vi "BLE_r&w.vi"() -> ()   [LabVIEW 2020]
uses:
  D:/Project/LabView/LabVIEW-BLE-Driver-main/BLE_base/BLELib.dll
  BLELib.dll
panel:
  out "错误输出":errorcluster
  out "StopResult":string
  out "添加的数组":u32[](array[numeric])
  out "NotifyResult":string
  out "Watcher Response":string
  in  "停止接收Notify":bool
  out "WriteResult":string
  out "NotifyStartResult":string
  out "目标设备地址":string
  in  "停止搜寻":bool
  out "蓝牙设备地址列表":string[][](array[string])
  out "设备搜寻状态":string
  in  "是否开启BLE蓝牙log日志":bool
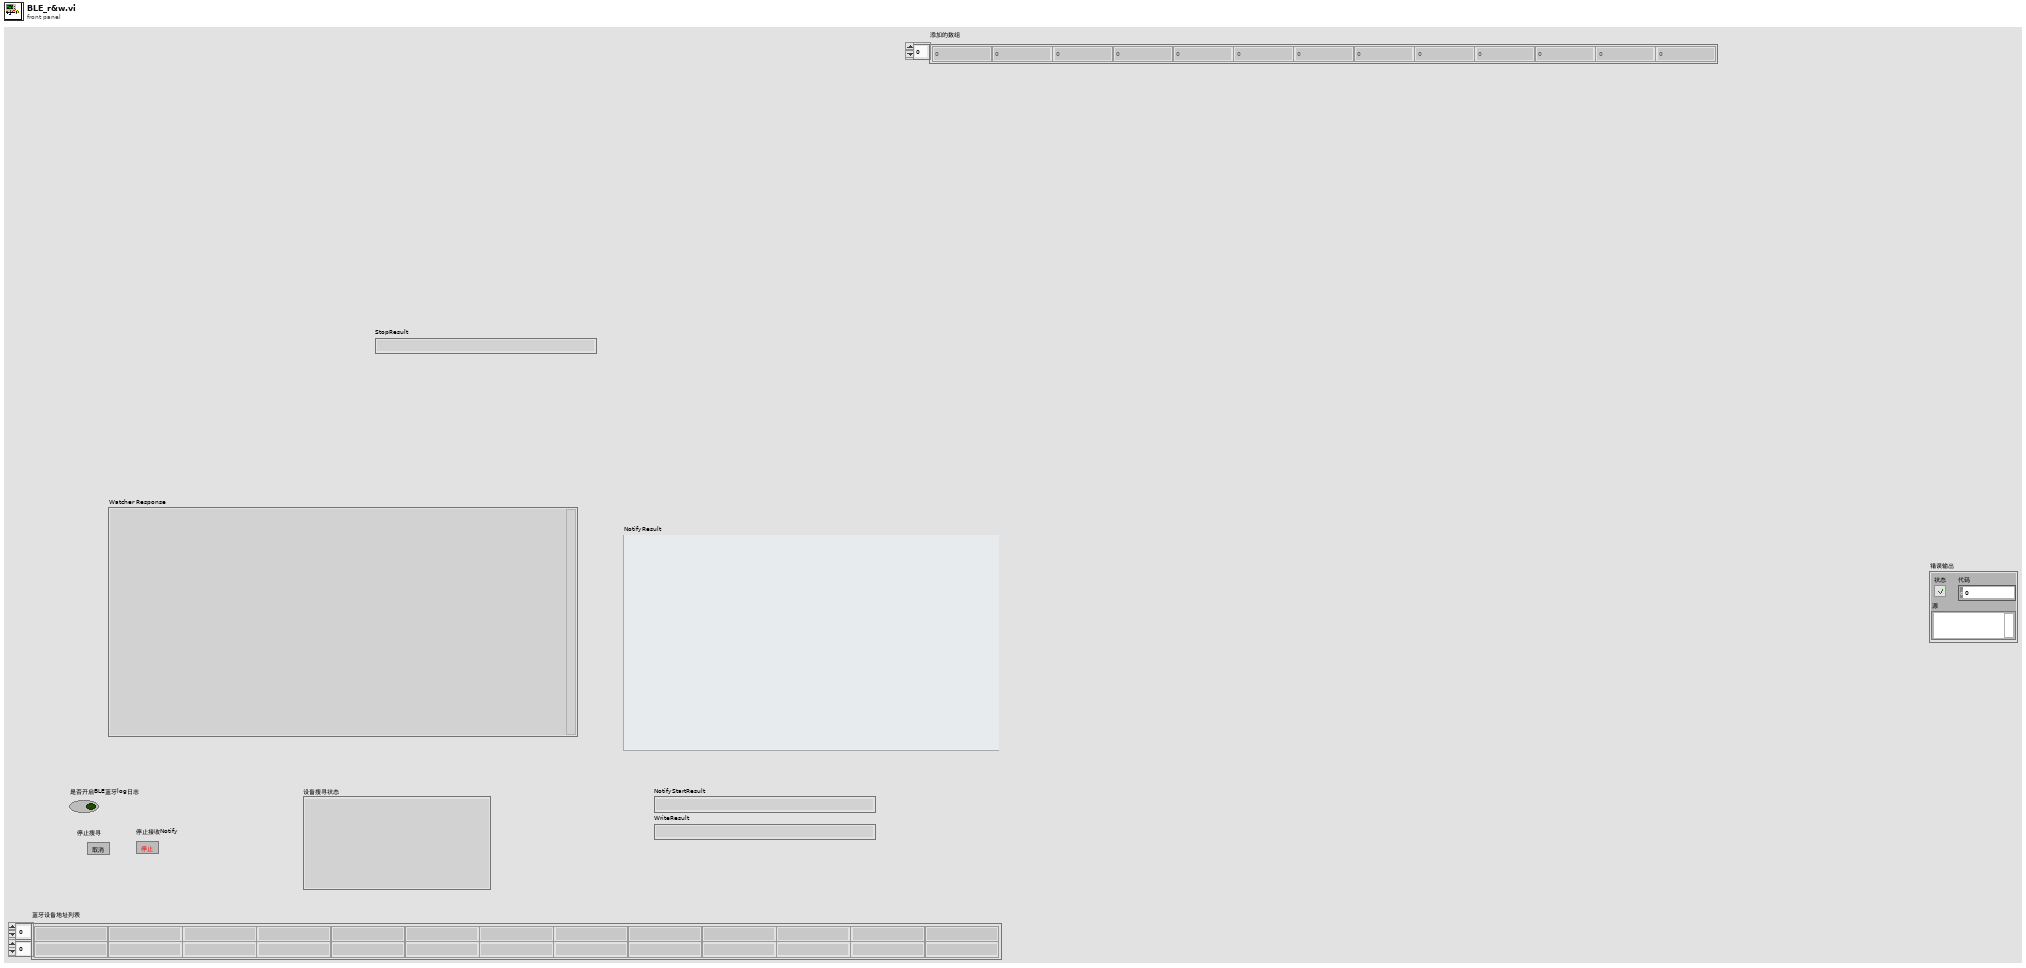
[diagram p1: front panel]
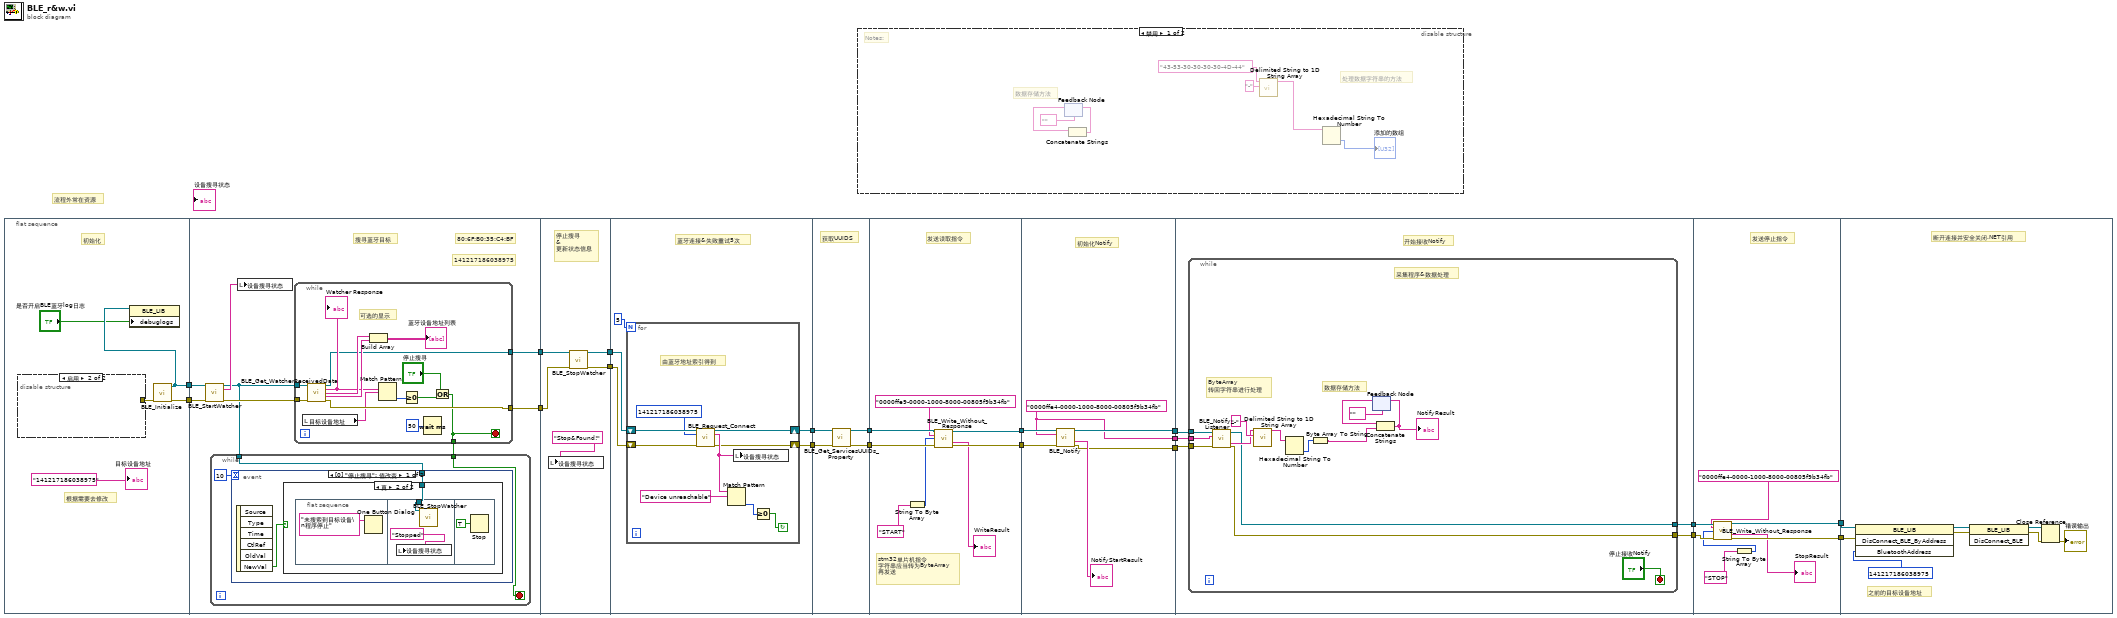
[diagram p0: block diagram]
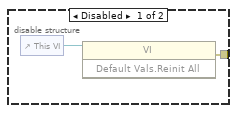
[diagram p3: hidden frame]
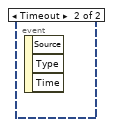
[diagram p5: hidden frame]
diagram:
  # "流程外常在资源"
  n1 = flat-sequence {
    tunnel: [w23] -> w19
    tunnel: [w21] -> w18
    tunnel: w19 -> [w34]
    tunnel: w18 -> [w33]
    tunnel: [w31] -> w17
    tunnel: [w30] -> w16
    tunnel: w17 -> [w62]
    tunnel: w16 -> [w60]
    tunnel: [w61] -> w15
    tunnel: [w59] -> w14
    tunnel: w15 -> [w67]
    tunnel: w14 -> [w66]
    tunnel: [w65] -> w13
    tunnel: [w64] -> w12
    tunnel: w13 -> [w81]
    tunnel: w12 -> [w80]
    tunnel: [w79] -> w11
    tunnel: [w78] -> w9
    tunnel: w11 -> [w89]
    tunnel: [w88] -> w10
    tunnel: w9 -> [w86]
    tunnel: [w87] -> w8
    tunnel: w10 -> [w95]
    tunnel: w8 -> [w94]
    tunnel: [w92] -> w7
    tunnel: [w91] -> w6
    tunnel: [w90] -> w5
    tunnel: w7 -> [w100]
    tunnel: w6 -> [w99]
    tunnel: w5 -> [w98]
    tunnel: [w97] -> w4
    tunnel: [w96] -> w3
    tunnel: w4 -> [w122]
    tunnel: w3 -> [w121]
    tunnel: [w117] -> w2
    tunnel: [w116] -> w1
    tunnel: w2 -> [w130]
    tunnel: w1 -> [w129]
    frame #0 {
      # "根据需要去修改"
      # "初始化"
      n2 = disable-structure shown="启用" {
        disable-tunnel: [w25 _] -> w24
        frame Disabled {
          n3 = control-ref of="This VI"() -> (w26:refnum<vi>)
          n4 = invoke class="VI" method="Default Vals.Reinit All"(reference=w26) -> (error out=w25:errorcluster)  [unwired: 2 in, 2 out]
        }
        frame Enabled {
        }
      }
      n5 = call "BLE_Initialize.vi"("error in (no error)"=w24) -> (".NET Refnum out"=w23:refnum<k24>, "error out"=w21:errorcluster)  [unwired: 13 in]
      n6 = property class="BLE_LIB"(reference=w23, "debuglogs"="是否开启BLE蓝牙log日志") -> ()  [unwired: 1 in, 2 out]
      "目标设备地址" <- "141217186038975" ("正则表达式")
    }
    frame #1 {
      # "141217186038975"
      # "80:6F:B0:35:C4:BF"
      # "搜寻蓝牙目标"
      n7 = call "BLE_StartWatcher.vi"(".NET Refnum in"=w34, "error in (no error)"=w33) -> (".NET Refnum out"=w28:refnum<k24>, "StartDeviceWatcher"=w29:string, "error out"=w32:errorcluster)  [unwired: 11 in]
      n8 = local write "设备搜寻状态"(w29) -> ()
      n9 = while {
        tunnel: w28 -> [w58]
        tunnel: w32 -> [w57]
        tunnel: [w49] -> w31
        tunnel: [w48] -> w30
        tunnel: [w46] -> w27
        stop <- w46 stop-if-true
        # "可选的显示"
        n10 = local read "目标设备地址"() -> (w47:string)
        n11 = call "BLE_Get_WatcherReceivedData.vi"(".NET Refnum in"=w58, "error in (no error)"=w57) -> (".NET Refnum out"=w49:refnum<k24>, "Watcher Response"=w53:string, "Bluetooth Addr"=w56:string[], "Bluetooth Raw Addr"=w55:string[], "error out"=w48:errorcluster)  [unwired: 6 in, 3 out]
        "Watcher Response" <- w53
        n12 = Build Array(w56, w55) -> (→"蓝牙设备地址列表":string[][])
        n13 = Match Pattern(string=w53, regular expression=w47) -> (offset past match=w52:i32)  [unwired: 1 in, 3 out]
        n14 = Greater Or Equal To 0?(x=w52) -> (x >= 0?=w51:bool)
        n15 = Wait (ms)(milliseconds to wait=u32 50 ("等待时间（毫秒）")) -> ()  [unwired: 1 out]
        n16 = Or(x="停止搜寻", y=w51) -> (x .or. y?=w46:bool)
      }
      n17 = while {
        tunnel: w28 -> [w37]
        tunnel: w27 -> [w36]
        stop <- w36 stop-if-true
        n18 = event shown="[0] \"停止搜寻\": 值改变" {
          selector: _ -> [_ _]
          dyn-events: _ -> [_ _]
          timeout: 10 -> [_ _]
          tunnel: w37 -> [w39 _]
          event "停止搜寻": Value Change {
            n19 = event-data() -> ("NewVal"=w38:bool)  [unwired: 1 in, 5 out]
            n20 = case shown="真" w38 {
              tunnel: w39 -> [_ w40]
              frame False {
              }
              frame True {
                n21 = flat-sequence {
                  tunnel: w40 -> [w43]
                  frame #0 {
                    n22 = One Button Dialog(message="未搜索到目标设备\n程序停止" ("消息")) -> ()  [unwired: 1 in, 1 out]
                  }
                  frame #1 {
                    n23 = local write "设备搜寻状态"("Stopped") -> ()
                    n24 = call "BLE_StopWatcher.vi"(".NET Refnum in"=w43) -> ()  [unwired: 12 in, 3 out]
                  }
                  frame #2 {
                    n25 = Stop(stop? (T)=TRUE ("停止？(T)")) -> ()
                  }
                }
              }
            }
          }
          event Timeout {
            n26 = event-data() -> ()  [unwired: 1 in, 3 out]
          }
        }
      }
    }
    frame #2 {
      # "停止搜寻\n&\n更新状态信息"
      n27 = local write "设备搜寻状态"("Stop&Found!") -> ()
      n28 = call "BLE_StopWatcher.vi"(".NET Refnum in"=w62, "error in (no error)"=w60) -> (".NET Refnum out"=w61:refnum<k24>, "error out"=w59:errorcluster)  [unwired: 11 in, 1 out]
    }
    frame #3 {
      # "蓝牙连接&失败重试5次"
      n29 = for {
        N: 5 -> [_]
        shift-right: [w70] -> w65
        shift-left: w67 -> [w77]
        shift-right: [w69] -> w64
        shift-left: w66 -> [w76]
        stop <- w71 continue-if-true
        # "由蓝牙地址索引得到"
        n30 = call "BLE_Request_Connect.vi"(".NET Refnum in"=w77, "BluetoothAddress"=u64 141217186038975, "error in (no error)"=w76) -> (".NET Refnum out"=w70:refnum<k24>, "ConnectBLE"=w74:string, "error out"=w69:errorcluster)  [unwired: 10 in]
        n31 = Match Pattern(string=w74, regular expression="Device unreachable") -> (offset past match=w72:i32)  [unwired: 1 in, 3 out]
        n32 = local write "设备搜寻状态"(w74) -> ()
        n33 = Greater Or Equal To 0?(x=w72) -> (x >= 0?=w71:bool)
      }
    }
    frame #4 {
      # "获取UUIDS"
      n34 = call "BLE_Get_ServicesUUIDs_Property.vi"(".NET Refnum in"=w81, "error in (no error)"=w80) -> (".NET Refnum out"=w79:refnum<k24>, "error out"=w78:errorcluster)  [unwired: 11 in, 1 out]
    }
    frame #5 {
      # "stm32单片机指令\n字符串应当转为ByteArray\n再发送"
      # "发送读取指令"
      n35 = String To Byte Array(string="START") -> (unsigned byte array=w83:u8[])
      n36 = call "BLE_Write_Without_Response.vi"(".NET Refnum in"=w89, "UUID"="0000ffe9-0000-1000-8000-00805f9b34fb", "WriteByteArray"=w83, "error in (no error)"=w86) -> (".NET Refnum out"=w88:refnum<k24>, "Result"=→"WriteResult":string, "error out"=w87:errorcluster)  [unwired: 9 in]
    }
    frame #6 {
      w90 = "0000ffe4-0000-1000-8000-00805f9b34fb" ("UUID")
      # "初始化Notify"
      n37 = call "BLE_Notify.vi"(".NET Refnum in"=w95, "UUID"=w90, "error in (no error)"=w94) -> (".NET Refnum out"=w92:refnum<k24>, "Result"=→"NotifyStartResult":string, "error out"=w91:errorcluster)  [unwired: 10 in]
    }
    frame #7 {
      # "开始接收Notify"
      n38 = while {
        tunnel: w100 -> [w114]
        tunnel: w99 -> [w113]
        tunnel: w98 -> [w112]
        tunnel: [w102] -> w97
        tunnel: [w101] -> w96
        stop <- "停止接收Notify" stop-if-true
        # "ByteArray\n转回字符串进行处理"
        # "采集程序&数据处理"
        # "数据存储方法"
        n39 = call "BLE_Notify_Listener.vi"(".NET Refnum in"=w114, "UUID"=w112, "error in (no error)"=w113) -> (".NET Refnum out"=w102:refnum<k24>, "Result"=w108:string, "error out"=w101:errorcluster)  [unwired: 10 in]
        n40 = call <vilib>:"Delimited String to 1D String Array.vi"("delimiter"="-", "delimited string"=w108) -> ("string array"=w110:string[])  [unwired: 9 in]
        n41 = Hexadecimal String To Number(string=w110) -> (number=w107:u32[])  [unwired: 2 in, 1 out]
        n42 = Byte Array To String(unsigned byte array=w107) -> (string=w104:string)
        n43 = feedback #1("") -> (w106:string)
        n44 = Concatenate Strings(w106, w104) -> (w103:string)
        "NotifyResult" <- w103
        n45 = feedback-in #1(w103) -> ()
      }
    }
    frame #8 {
      # "发送停止指令"
      n46 = String To Byte Array(string="STOP") -> (unsigned byte array=w118:u8[])
      n47 = call "BLE_Write_Without_Response.vi"(".NET Refnum in"=w122, "UUID"="0000ffe4-0000-1000-8000-00805f9b34fb", "WriteByteArray"=w118, "error in (no error)"=w121) -> (".NET Refnum out"=w117:refnum<k24>, "Result"=→"StopResult":string, "error out"=w116:errorcluster)  [unwired: 9 in]
    }
    frame #9 {
      # "断开连接并安全关闭.NET引用"
      # "之前的目标设备地址"
      n48 = invoke on="调用节点" class="BLE_LIB" method="DisConnect_BLE_ByAddress"(reference=w130, error in=w129, "BluetoothAddress"=u64 141217186038975) -> (reference out=w127:refnum<k24>, error out=w126:errorcluster)  [unwired: 1 in, 2 out]
      n49 = invoke on="调用节点" class="BLE_LIB" method="DisConnect_BLE"(reference=w127, error in=w126) -> (reference out=w124:refnum<k24>, error out=w123:errorcluster)  [unwired: 1 in, 1 out]
      n50 = Close Reference(reference=w124, error in (no error)=w123) -> (error out=→"错误输出":errorcluster)
    }
  }
  n51 = disable-structure shown="禁用" {
    frame Disabled {
      # "Notes:"
      # "数据存储方法"
      # "处理数据字符串的方法"
      n52 = feedback #2("") -> (w132:string)
      n53 = Concatenate Strings(w132) -> (w134:string, w133:string)
      n54 = feedback-in #2(w134) -> ()
      n55 = call <vilib>:"Delimited String to 1D String Array.vi"("delimiter"="-", "delimited string"="43-53-30-30-30-30-4D-44") -> ("string array"=w136:string[])  [unwired: 9 in]
      n56 = Hexadecimal String To Number(string=w136) -> (number=→"添加的数组":u32[])  [unwired: 2 in, 1 out]
    }
    frame Enabled {
    }
  }
